vi "Initialize.vi"(8 "Error In":errorcluster, 11 "TopLevel In":T1) -> (0 "Error Out":errorcluster, 3 "TopLevel Out":T1)   [LabVIEW 2011]
uses:
  Controls/Top Level Control.ctl
  <vilib>/NI/AMC/Message Queue.ctl
  <vilib>/NI/AMC/Message.ctl
  <vilib>/NI/Tools/Keyed Array/KeyedArray.ctl
  Controls/ListBox Test Record.ctl
  Controls/DVR of CSV Tests Data.ctl
  Controls/CSVs Tests Data.ctl
  Controls/Test Column Data.ctl
  Controls/Options DVR.ctl
  Controls/Options.ctl
  <vilib>/NI/AMC/AMC.lvlib
  <vilib>/NI/Tools/Keyed Array/Tools_KeyedArray.lvlib
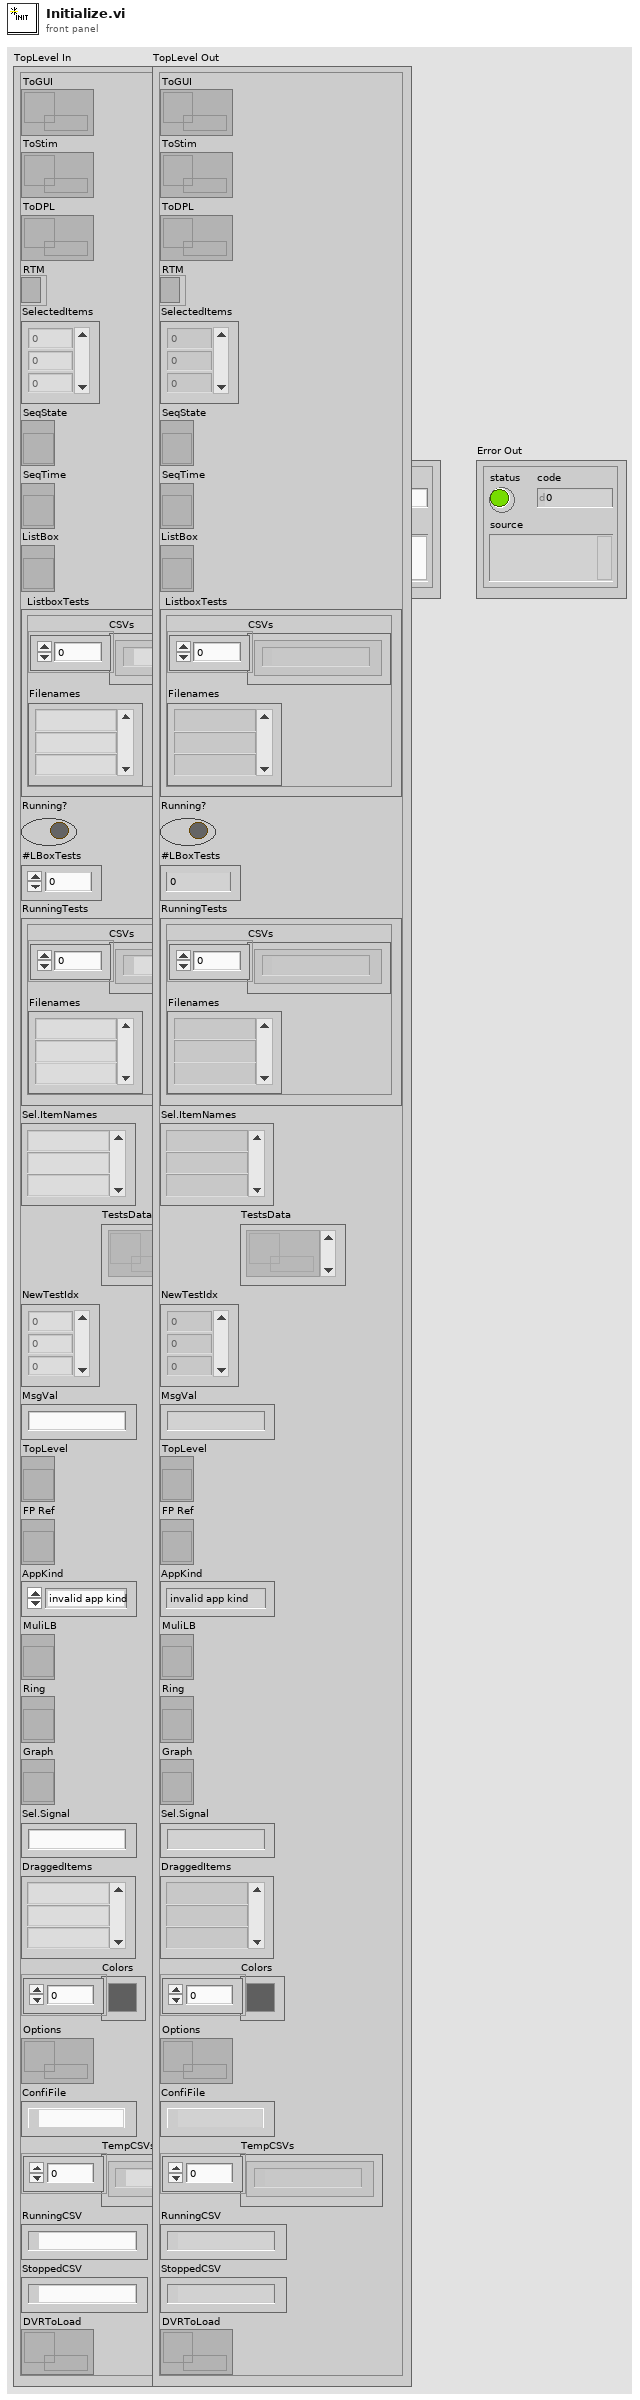
[diagram p1: front panel]
types:
  T1 = typedef "Top Level Control.ctl" = cluster{"ToGUI":T2, "ToStim":T2, "ToDPL":T2, "RTM":refnum<k9>, "SelectedItems":i32[], "SeqState":refnum<vi>, "SeqTime":refnum<vi>, "ListBox":refnum<vi>, "ListboxTests":T3, "Running?":bool, "#LBoxTests":i32, "RunningTests":T3, "Sel.ItemNames":string[], "TestsData":T4[], "NewTestIdx":i32[], "MsgVal":string, "TopLevel":refnum<vi>, "FP Ref":refnum<vi>, "AppKind":enum32{"invalid app kind", "Development System", "Run Time System", "Student Edition", "Embedded LabVIEW", "Evaluation", "Custom"}, "MuliLB":refnum<vi>, "Ring":refnum<vi>, "Graph":refnum<vi>, "Sel.Signal":string, "DraggedItems":string[], "Colors":u32[], "Options":T5, "ConfiFile":path, "TempCSVs":path[], "RunningCSV":path, "StoppedCSV":path, "DVRToLoad":T4}
  T2 = typedef "AMC.lvlib/Message Queue.ctl" = refnum<queue>
  T3 = typedef "ListBox Test Record.ctl" = cluster{"CSVs":path[], "Filenames":string[]}
  T4 = typedef "DVR of CSV Tests Data.ctl" = refnum<data-value>
  T5 = typedef "Options DVR.ctl" = refnum<data-value>
  T6 = enum32{"invalid app kind", "Development System", "Run Time System", "Student Edition", "Embedded LabVIEW", "Evaluation", "Custom"}
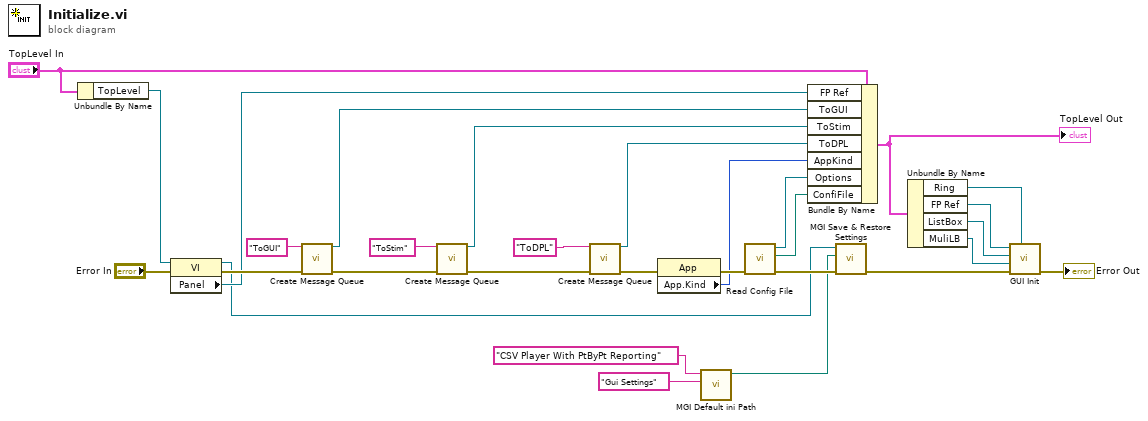
[diagram p0: block diagram]
diagram:
  n1 = Unbundle By Name("TopLevel In") -> ("TopLevel"=w22:refnum<vi>)
  n2 = property class="VI"(reference=w22, error in="Error In") -> (reference out=w4:refnum<vi>, error out=w21:errorcluster, "Panel"=w20:refnum<vi>)
  n3 = call <vilib>:"Create Message Queue.vi"("message queue name"="ToGUI" ("Message Queue Name"), "error in"=w21) -> ("message queue out"=w25:T2, "error out"=w30:errorcluster)  [unwired: 12 in]
  n4 = call <vilib>:"Create Message Queue.vi"("message queue name"="ToStim" ("Message Queue Name"), "error in"=w30) -> ("message queue out"=w24:T2, "error out"=w29:errorcluster)  [unwired: 12 in]
  n5 = call <vilib>:"Create Message Queue.vi"("message queue name"="ToDPL" ("Message Queue Name"), "error in"=w29) -> ("message queue out"=w23:T2, "error out"=w19:errorcluster)  [unwired: 12 in]
  n6 = property class="App"(error in=w19) -> (error out=w18:errorcluster, "App.Kind"=w8:T6)  [unwired: 1 in, 1 out]
  n7 = call <userlib>:"MGI Default ini Path.vi"("File Name (Caller's Prefix)"="Gui Settings", "Folder Name (Caller's Prefix)"="CSV Player With PtByPt Reporting") -> ("Path"=w1:path)  [unwired: 9 in]
  n8 = call "Read Config File.vi"("error in (no error)"=w18) -> ("error out"=w6:errorcluster, "ConfigFile"=w7:path, "Data Value Reference out"=w17:T5)  [unwired: 8 in]
  n9 = Bundle By Name(cluster="TopLevel In", "FP Ref"=w20, "ToGUI"=w25, "ToStim"=w24, "ToDPL"=w23, "AppKind"=w8, "Options"=w17, "ConfiFile"=w7) -> (w9:T1)
  "TopLevel Out" <- w9
  n10 = call <userlib>:"MGI Save & Restore Settings.vi"("Error In"=w6, "Path"=w1, "VI Reference In (Caller)"=w4) -> ("Error Out"=w5:errorcluster)  [unwired: 7 in, 1 out]
  n11 = Unbundle By Name(w9) -> ("Ring"=w15:refnum<vi>, "FP Ref"=w14:refnum<vi>, "ListBox"=w13:refnum<vi>, "MuliLB"=w12:refnum<vi>)
  n12 = call "GUI Init.vi"("Ring"=w15, "error in (no error)"=w5, "MuliLB"=w12, "ListBox"=w13, "FP Ref"=w14) -> ("error out"=→"Error Out":errorcluster)  [unwired: 6 in]
